vi "4_6.vi"() -> ()   [LabVIEW 2017]
panel:
  out "Cluster":T1
  out "Waveform Chart  (Sweep)":dbl(graph)
  out "Waveform Chart (Strip)":dbl(graph)
  in  "stop":bool
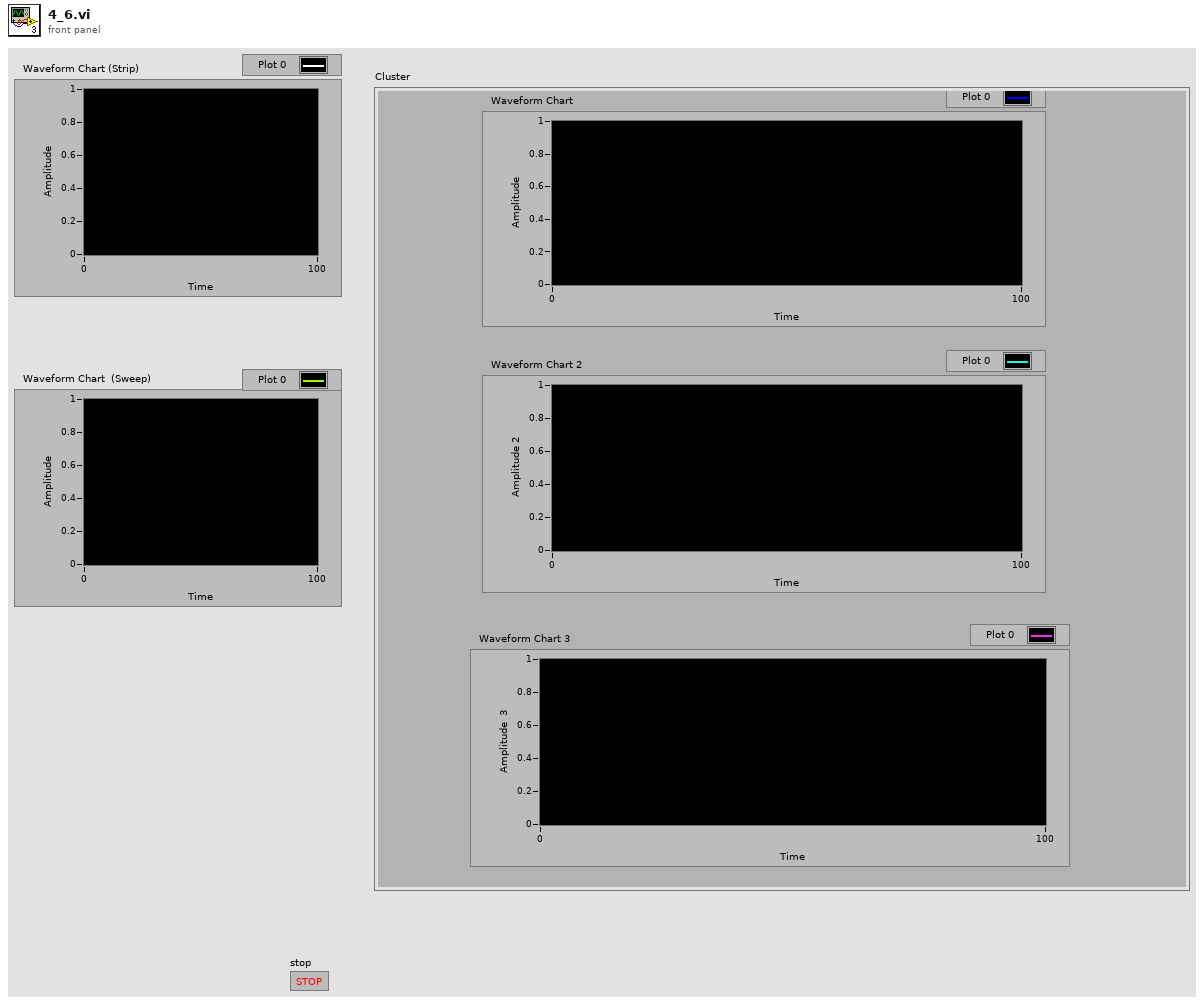
[diagram p1: front panel]
types:
  T1 = cluster{"Waveform Chart":dbl, "Waveform Chart 2":dbl, "Waveform Chart 3":dbl}
  T2 = cluster{"number: 0 to 1":dbl, "number: 0 to 1":dbl, "number: 0 to 1":dbl}
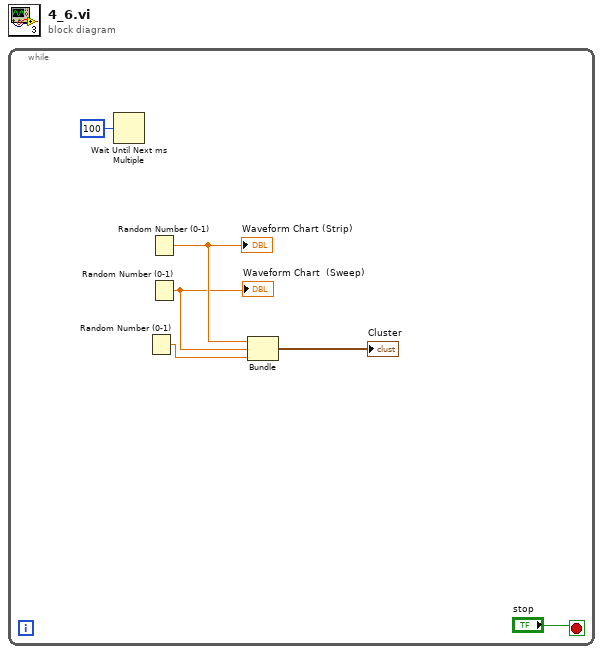
[diagram p0: block diagram]
diagram:
  n1 = while {
    stop <- "stop" stop-if-true
    n2 = Wait Until Next ms Multiple(millisecond multiple=u32 100) -> ()  [unwired: 1 out]
    n3 = Random Number (0-1)() -> (number: 0 to 1=w2:dbl)
    n4 = Random Number (0-1)() -> (number: 0 to 1=w4:dbl)
    "Waveform Chart (Strip)" <- w4
    n5 = Random Number (0-1)() -> (number: 0 to 1=w3:dbl)
    "Waveform Chart  (Sweep)" <- w3
    n6 = Bundle("number: 0 to 1"=w4, "number: 0 to 1"=w3, "number: 0 to 1"=w2) -> (→"Cluster":T2)  [unwired: 1 in]
  }
